vi "iWorx - Heart Sounds.vi"() -> ()   [LabVIEW 2012]
uses:
  vi.lib/iWorx/iWorx Set Points.ctl
  <vilib>/DAQmx/create/channels.llb/DAQmx Create Channel (AI-Voltage-Basic).vi
  <vilib>/DAQmx/configure/timing.llb/DAQmx Timing (Sample Clock).vi
  <vilib>/DAQmx/read.llb/DAQmx Read (Analog 1D Wfm NChan 1Samp).vi
panel:
  in  "Reset Scale":bool
  in  "Stop":bool
  in  "Log Info Button":bool
  in  "Set Up":bool
  in  "Channel":u16(ring) items=["Channel 1", "Channel 2"]
  in  "Pause Button":bool
  in  "Snapshot":bool
  out "Processed Signal":dbl(knob) caption="Pressue" scale=0.0..20.0
  out "Waveform Chart":waveform(dbl)(graph)
  in  "Clear Chart":bool
  in  "Open Log":bool
  in  "Rescale Y":bool
  out "Raw Signal":dbl(knob) scale=-10.0..10.0
  # "iWorx - Heart Sounds - Data Logger"
  # "Sensor Input"
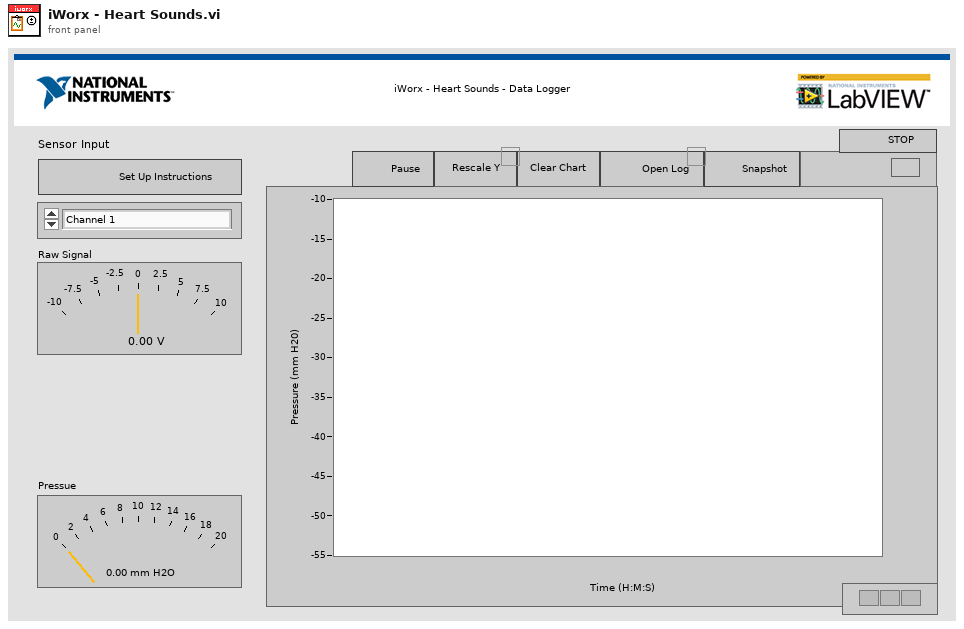
[diagram p1: front panel]
types:
  T1 = typedef "iWorx Set Points.ctl" = cluster{"SP1 Voltage":dbl, "SP1 Value":dbl, "SP2 Voltage":dbl, "SP2 Value":dbl}
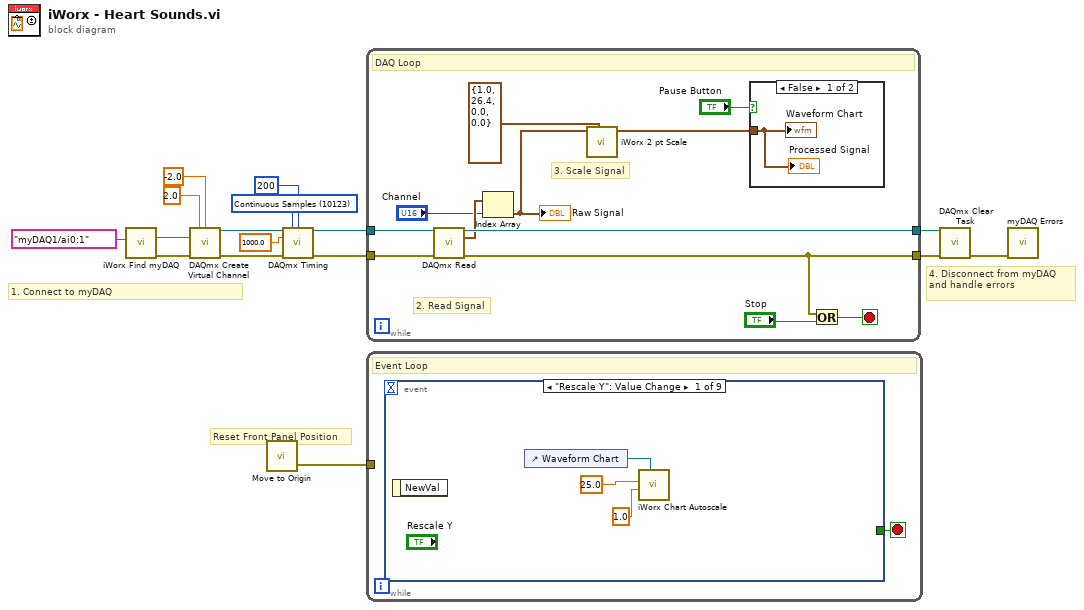
[diagram p0: block diagram]
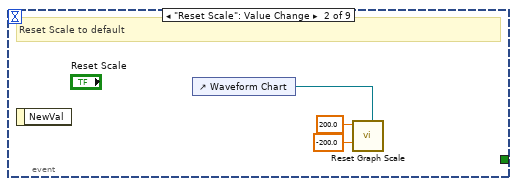
[diagram p2: hidden frame]
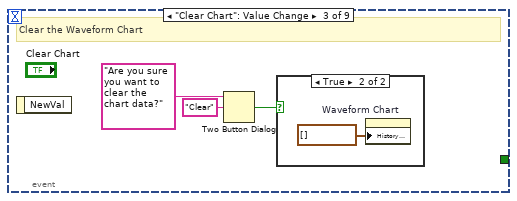
[diagram p3: hidden frame]
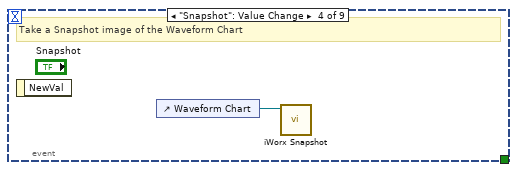
[diagram p5: hidden frame]
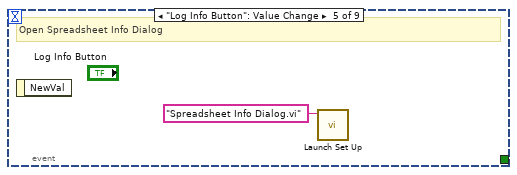
[diagram p6: hidden frame]
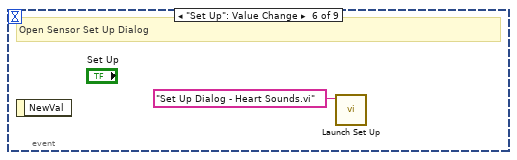
[diagram p7: hidden frame]
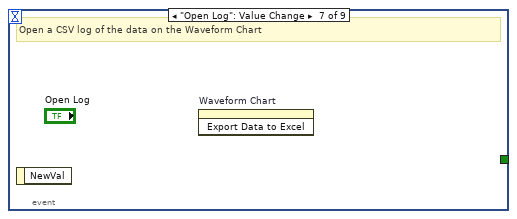
[diagram p8: hidden frame]
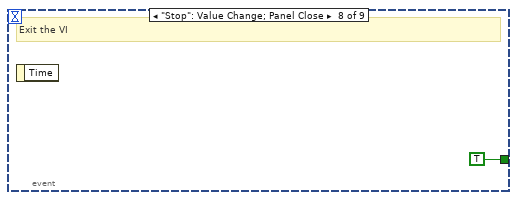
[diagram p9: hidden frame]
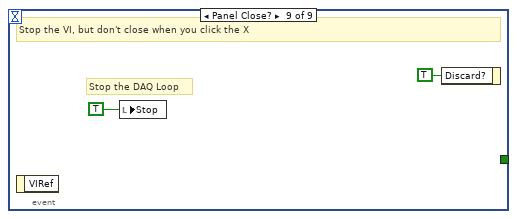
[diagram p10: hidden frame]
diagram:
  w7 = 10123 items=["Finite Samples"=10178, "Continuous Samples"=10123, "Hardware Timed Single Point"=12522] ("sample mode")
  # "Reset Front Panel Position"
  # "4. Disconnect from myDAQ and handle errors"
  # "1. Connect to myDAQ"
  n1 = call "iWorx Find myDAQ.vi"("Preferred myDAQ (myDAQ1)"=tag "myDAQ1/ai0:1") -> ("Error Out"=w12:errorcluster, "DAQmx Physical Channel"=w13:tag)  [unwired: 6 in, 3 out]
  n2 = call-poly <vilib>:"DAQmx Create Virtual Channel.vi"("maximum value"=2.0, "minimum value"=-2.0, "physical channels"=w13, "error in"=w12) -> ("task out"=w5:refnum<k21>, "error out"=w2:errorcluster)  [unwired: 10 in]
  n3 = call "Move to Origin.vi"() -> ("Error Out"=w10:errorcluster)  [unwired: 3 in]
  n4 = call-poly <vilib>:"DAQmx Timing.vi"("task/channels in"=w5, "sample mode"=w7, "samples per channel"=200, "rate"=1000.0, "error in"=w2) -> ("task out"=w4:refnum<k21>, "error out"=w3:errorcluster)  [unwired: 9 in]
  n5 = while {
    tunnel: w4 -> [w28]
    tunnel: [w27] -> w16
    tunnel: w3 -> [w26]
    tunnel: [w24] -> w15
    stop <- w25 stop-if-true
    # "3. Scale Signal"
    # "2. Read Signal"
    # "DAQ Loop"
    n6 = call-poly <vilib>:"DAQmx Read.vi"("task/channels in"=w28, "error in"=w26) -> ("task out"=w27:refnum<k21>, "data"=w22:waveform(dbl)[], "error out"=w24:errorcluster)  [unwired: 11 in]
    n7 = Index Array(array=w22, index="Channel") -> (element=w20:waveform(dbl))
    "Raw Signal" <- w20
    n8 = call "iWorx 2 pt Scale.vi"("Set Points"=T1 {"SP1 Voltage"=1.0, "SP1 Value"=26.4, "SP2 Voltage"=0.0, "SP2 Value"=0.0}, "Raw Waveform"=w20) -> ("Scaled Value"=w21:waveform(dbl))  [unwired: 7 in, 2 out]
    n9 = case shown="False" "Pause Button" {
      tunnel: w21 -> [w29 _]
      frame False {
        "Waveform Chart" <- w29
        "Processed Signal" <- w29
      }
      frame True {
        # "Do Not update controls"
      }
    }
    n10 = Or(x=w24, y="Stop") -> (x .or. y?=w25:bool)
  }
  n11 = while {
    tunnel: w10 -> [_]
    stop <- w30 stop-if-true
    # "Event Loop"
    n12 = event shown="[0] \"Rescale Y\": Value Change" {
      selector: _ -> [_ _ _ _ _ _ _ _ _]
      dyn-events: _ -> [_ _ _ _ _ _ _ _ _]
      timeout: _ -> [_ _ _ _ _ _ _ _ _]
      tunnel: [_ _ _ _ _ _ _ TRUE _] -> w30
      event "Rescale Y": Value Change {
        n13 = event-data() -> ()  [unwired: 1 in, 1 out]
        n14 = control-ref of="Waveform Chart"() -> (w33:refnum<vi>)
        n15 = call "iWorx Chart Autoscale.vi"("Selection Chart"=w33, "Rounding Multiple (10)"=1.0 ("Rounding Multiple (1)"), "Padding (10%)"=25.0 ("Rounding Multiple (1)")) -> ()  [unwired: 6 in, 3 out]
      }
      event "Reset Scale": Value Change {
        # "Reset Scale to default"
        n16 = event-data() -> ()  [unwired: 1 in, 1 out]
        n17 = control-ref of="Waveform Chart"() -> (w36:refnum<vi>)
        n18 = call "Reset Graph Scale.vi"("WaveformChart in"=w36, "Minimum (0)"=-200.0, "Maximum (100)"=200.0) -> ()  [unwired: 9 in]
      }
      event "Clear Chart": Value Change {
        # "Clear the Waveform Chart"
        n19 = event-data() -> ()  [unwired: 1 in, 1 out]
        n20 = Two Button Dialog(message="Are you sure you want to clear the chart data?", 2:"Clear" ("T button name (\"OK\")")) -> (T button?=w38:bool)  [unwired: 1 in]
        n21 = case shown="True" w38 {
          frame False {
          }
          frame True {
            n22 = property on="Waveform Chart" class="WFChart (strict)"("History Data"=waveform(dbl)[] []) -> ()  [unwired: 2 in, 2 out]
          }
        }
      }
      event "Snapshot": Value Change {
        # "Take a Snapshot image of the Waveform Chart"
        n23 = event-data() -> ()  [unwired: 1 in, 1 out]
        n24 = control-ref of="Waveform Chart"() -> (w41:refnum<vi>)
        n25 = call "iWorx Snapshot.vi"("WaveformChart in"=w41) -> ()  [unwired: 10 in, 1 out]
      }
      event "Log Info Button": Value Change {
        # "Open Spreadsheet Info Dialog"
        n26 = event-data() -> ()  [unwired: 1 in, 1 out]
        n27 = call "Launch Set Up.vi"("name or relative path"="Spreadsheet Info Dialog.vi") -> ()  [unwired: 9 in, 2 out]
      }
      event "Set Up": Value Change {
        # "Open Sensor Set Up Dialog"
        n28 = event-data() -> ()  [unwired: 1 in, 1 out]
        n29 = call "Launch Set Up.vi"("name or relative path"="Set Up Dialog - Heart Sounds.vi") -> ()  [unwired: 9 in, 2 out]
      }
      event "Open Log": Value Change {
        # "Open a CSV log of the data on the Waveform Chart"
        n30 = event-data() -> ()  [unwired: 1 in, 1 out]
        n31 = invoke on="Waveform Chart" class="WFChart (strict)" method="Export Data to Excel"() -> ()  [unwired: 3 in, 3 out]
      }
      event "Stop": Value Change; Panel Close {
        # "Exit the VI"
        n32 = event-data() -> ()  [unwired: 1 in, 1 out]
      }
      event Panel Close? {
        # "Stop the DAQ Loop"
        # "Stop the VI, but don't close when you click the X"
        n33 = event-data() -> ()  [unwired: 1 in, 1 out]
        n34 = local write "Stop"(TRUE ("stop")) -> ()
        n35 = event-data("Discard?"=TRUE) -> ()  [unwired: 1 in, 1 out]
      }
    }
  }
  n36 = call <vilib>:"DAQmx Clear Task.vi"("task in"=w16, "error in"=w15) -> ("error out"=w14:errorcluster)  [unwired: 13 in]
  n37 = call "myDAQ Errors.vi"("error in (no error)"=w14) -> ()  [unwired: 10 in, 1 out]
